vi "UiMonitor.vi"() -> ()   [LabVIEW 2011]
panel:
  in  "Input Var":refnum<k21>="ni.var.psp://10.27.40.24/variables - b2g1/input - network b2g1"
  in  "Output Var":refnum<k21>="ni.var.psp://10.27.40.24/variables - b2g1/data - network - b2g1"
  in  "stop":bool
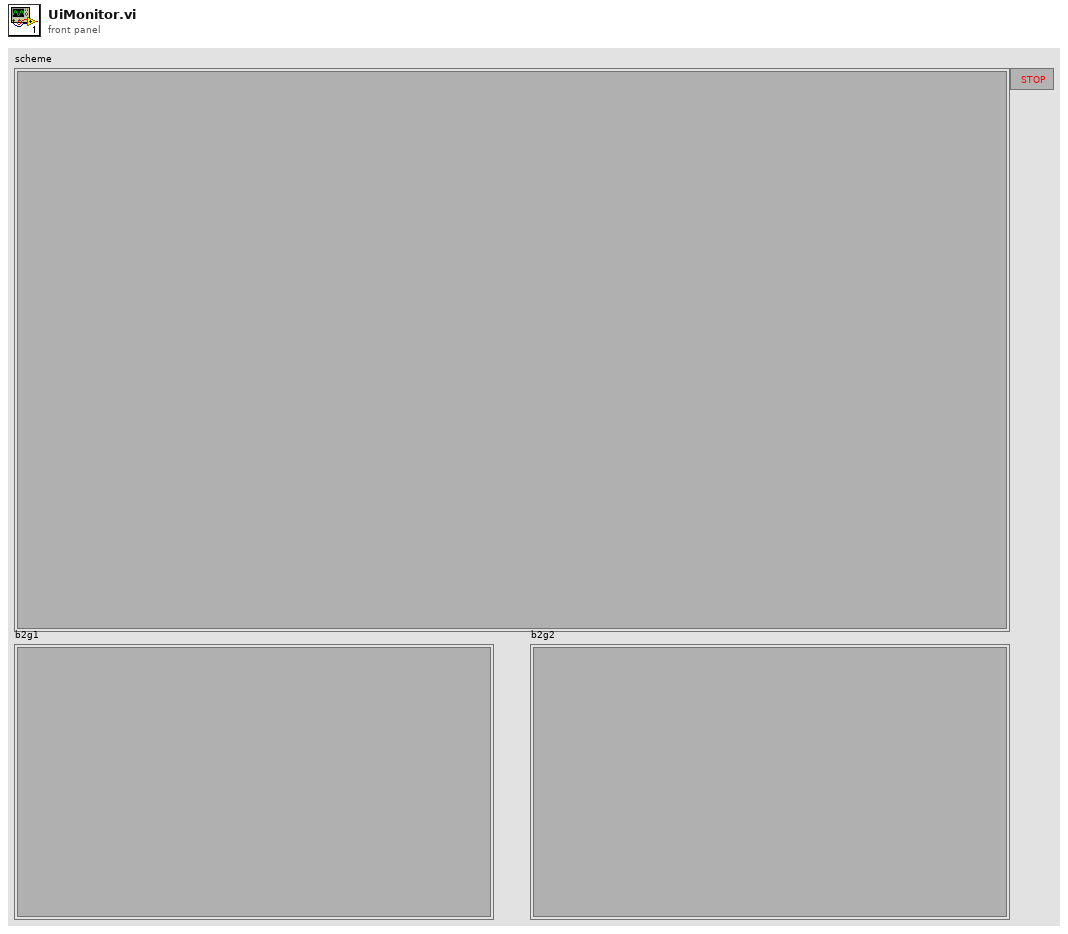
[diagram p1: front panel]
types:
  T1 = enum16{"Always On", "Always Off", "Off While Running"}
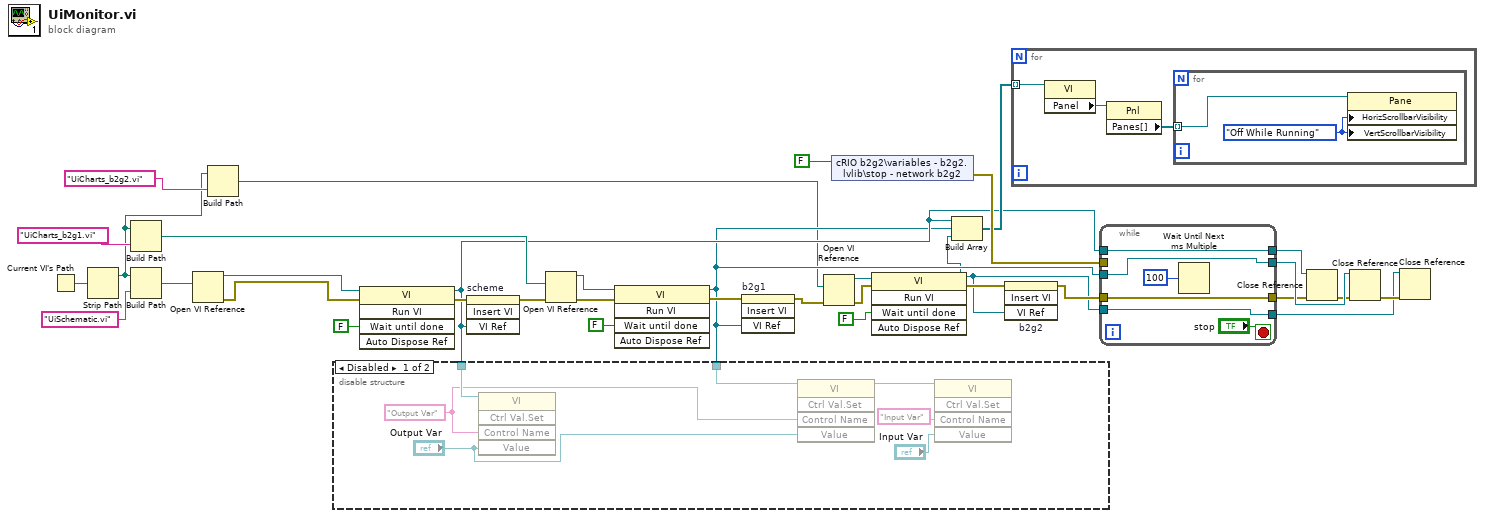
[diagram p0: block diagram]
diagram:
  n1 = Current VI's Path() -> (path=w22:path)
  n2 = Strip Path(path=w22) -> (stripped path=w5:path)  [unwired: 1 out]
  n3 = Build Path(base path=w5, name or relative path="UiCharts_b2g1.vi") -> (appended path=w27:path)
  n4 = Build Path(base path=w5, name or relative path="UiSchematic.vi") -> (appended path=w30:path)
  n5 = Open VI Reference(vi path=w30) -> (vi reference=w19:refnum<vi>, error out=w18:errorcluster)  [unwired: 5 in]
  n6 = Build Path(base path=w5, name or relative path="UiCharts_b2g2.vi") -> (appended path=w12:path)
  n7 = invoke class="VI" method="Run VI"(reference=w19, error in=w18, "Wait until done"=FALSE) -> (reference out=w17:refnum<vi>, error out=w32:errorcluster)  [unwired: 2 in, 3 out]
  n8 = invoke on="scheme" class="SubPanel" method="Insert VI"(error in=w32, "VI Ref"=w17) -> (error out=w24:errorcluster)  [unwired: 2 in, 3 out]
  n9 = Open VI Reference(vi path=w27, error in (no error)=w24) -> (vi reference=w16:refnum<vi>, error out=w15:errorcluster)  [unwired: 4 in]
  n10 = invoke class="VI" method="Run VI"(reference=w16, error in=w15, "Wait until done"=FALSE) -> (reference out=w14:refnum<vi>, error out=w26:errorcluster)  [unwired: 2 in, 3 out]
  n11 = disable-structure shown="Disabled" {
    disable-tunnel: w17 -> [w38 _]
    disable-tunnel: w14 -> [w37 _]
    frame Disabled {
      w36 = "Output Var" ("Control Name")
      n12 = invoke class="VI" method="Ctrl Val.Set"(reference=w38, "Control Name"=w36, "Value"="Output Var") -> ()  [unwired: 2 in, 5 out]
      n13 = invoke class="VI" method="Ctrl Val.Set"(reference=w37, "Control Name"=w36, "Value"="Output Var") -> (reference out=w40:refnum<vi>)  [unwired: 2 in, 4 out]
      n14 = invoke class="VI" method="Ctrl Val.Set"(reference=w40, "Control Name"="Input Var", "Value"="Input Var") -> ()  [unwired: 2 in, 5 out]
    }
    frame Enabled {
    }
  }
  n15 = invoke on="b2g1" class="SubPanel" method="Insert VI"(error in=w26, "VI Ref"=w14) -> (error out=w7:errorcluster)  [unwired: 2 in, 3 out]
  n16 = Open VI Reference(vi path=w12, error in (no error)=w7) -> (vi reference=w11:refnum<vi>, error out=w6:errorcluster)  [unwired: 4 in]
  n17 = shared-variable "cRIO b2g2\\variables - b2g2.lvlib\\stop - network b2g2"(FALSE ("stop - network")) -> (error out=w35:errorcluster)  [unwired: 1 in]
  n18 = invoke class="VI" method="Run VI"(reference=w11, error in=w6, "Wait until done"=FALSE) -> (reference out=w2:refnum<vi>, error out=w4:errorcluster)  [unwired: 2 in, 3 out]
  n19 = Build Array(w17, w14, w2) -> (w21:refnum<vi>[])
  n20 = invoke on="b2g2" class="SubPanel" method="Insert VI"(error in=w4, "VI Ref"=w2) -> (error out=w3:errorcluster)  [unwired: 2 in, 3 out]
  n21 = for {
    tunnel: w21 -> [w44] mode=indexing
    n22 = property class="VI"(reference=w44) -> ("Panel"=w43:refnum<vi>)  [unwired: 1 in, 2 out]
    n23 = property class="Pnl"(reference=w43) -> ("Panes[]"=w45:refnum<vi>[])  [unwired: 1 in, 2 out]
    n24 = for {
      tunnel: w45 -> [w47] mode=indexing
      w46 = T1."Off While Running" ("Scrollbar Visibility")
      n25 = property class="Pane"(reference=w47, "HorizScrollbarVisibility"=w46, "VertScrollbarVisibility"=w46) -> ()  [unwired: 1 in, 2 out]
    }
  }
  n26 = while {
    tunnel: w35 -> [_]
    tunnel: [w51] -> w31
    tunnel: w17 -> [w51]
    tunnel: w14 -> [w50]
    tunnel: [w50] -> w25
    tunnel: [w49] -> w20
    tunnel: w3 -> [w49]
    tunnel: w2 -> [w48]
    tunnel: [w48] -> w8
    stop <- "stop" stop-if-true
    n27 = Wait Until Next ms Multiple(millisecond multiple=u32 100) -> ()  [unwired: 1 out]
  }
  n28 = Close Reference(reference=w31, error in (no error)=w20) -> (error out=w23:errorcluster)
  n29 = Close Reference(reference=w25, error in (no error)=w23) -> (error out=w9:errorcluster)
  n30 = Close Reference(reference=w8, error in (no error)=w9) -> ()  [unwired: 1 out]
